vi "Duel Speed Ramp.vi"(6 "Total Distance":dbl, 8 "Current Distance":dbl, 9 "Distance":dbl, 10 "End":dbl, 11 "Start":dbl) -> (3 "Speed":dbl)   [LabVIEW 2016]
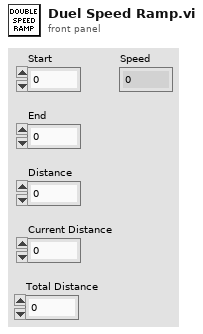
[diagram p1: front panel]
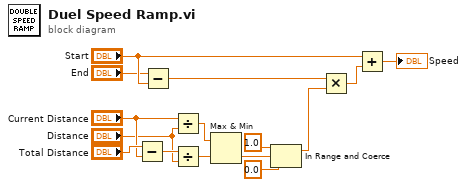
[diagram p0: block diagram]
diagram:
  n1 = Subtract(x="Total Distance", y="Current Distance") -> (x-y=w8:dbl)
  n2 = Subtract(x="End", y="Start") -> (x-y=w12:dbl)
  n3 = Divide(x="Current Distance", y="Distance") -> (x/y=w6:dbl)
  n4 = Divide(x=w8, y="Distance") -> (x/y=w5:dbl)
  n5 = Max & Min(x=w6, y=w5) -> (min(x,y)=w4:dbl)  [unwired: 1 out]
  n6 = In Range and Coerce(upper limit=1.0, x=w4, lower limit=0.0) -> (coerced(x)=w1:dbl)  [unwired: 1 out]
  n7 = Multiply(x=w12, y=w1) -> (x*y=w13:dbl)
  n8 = Add(x="Start", y=w13) -> (x+y=→"Speed":dbl)
